vi "Write Class fp.vi"(8 "error in":errorcluster, 10 "Class fp":path, 11 "Client in":refnum<class "Client.lvclass">) -> (0 "error out":errorcluster, 3 "Client out":refnum<class "Client.lvclass">)   [LabVIEW 2014, in "Client.lvclass"]
uses:
  Client.lvclass
  Client.lvclass/Client.ctl
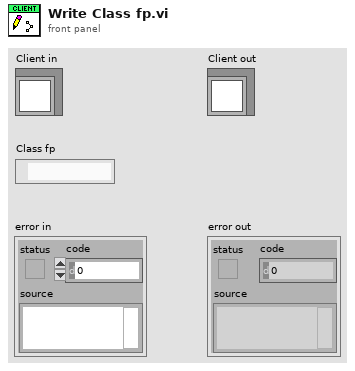
[diagram p1: front panel]
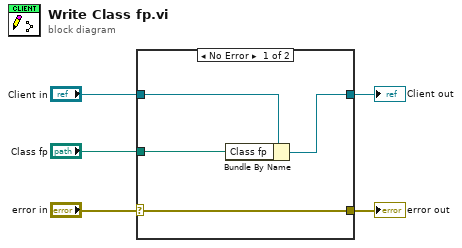
[diagram p0: block diagram]
diagram:
  n1 = case shown="No Error" "error in" {
    selector: "error in" -> [w9 w10]
    tunnel: [w9 w10] -> w4
    tunnel: [w7 w11] -> w2
    tunnel: "Client in" -> [w8 w11]
    tunnel: "Class fp" -> [w6 _]
    frame No Error {
      n2 = Bundle By Name(cluster=w8, "Class fp"=w6) -> (w7:refnum<class "Client.lvclass">)
    }
    frame Error {
    }
  }
  "error out" <- w4
  "Client out" <- w2
